vi "test list shell.vi"() -> ()   [LabVIEW 2014]
panel:
  out "Numeric":i32
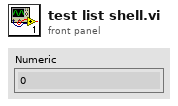
[diagram p1: front panel]
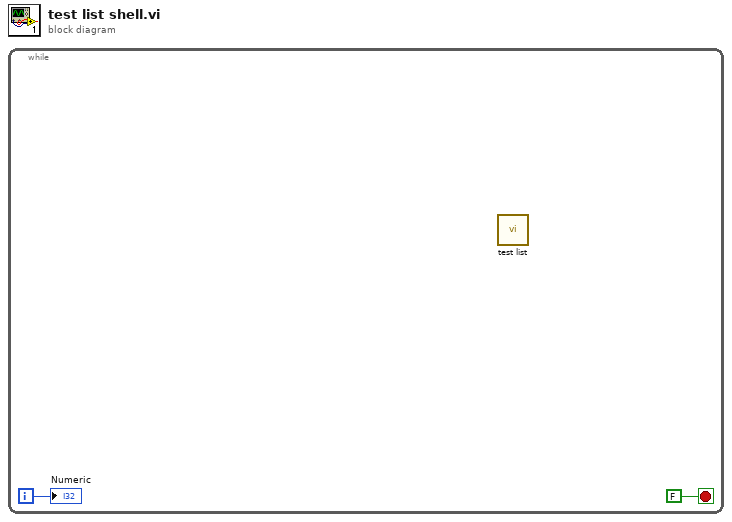
[diagram p0: block diagram]
diagram:
  n1 = while {
    i -> [w1]
    stop <- FALSE stop-if-true
    n2 = call "test list.vi"() -> ()  [unwired: 12 in]
    "Numeric" <- w1
  }
